vi "Coefficients for Exponential Averaging.vi"(2 "sampling frequency [Hz]":dbl=10000.0 format="%.2f", 3 "time constant [ms]":dbl=125.0 min=0.0 format="%.2f", 4 "exponential mode":enum16{"Slow", "Fast", "Impulse", "Custom"}(ring)=enum."Fast") -> (0 "actual time constant [ms]":dbl=125.0 format="%.2f", 1 "filter coefficients":T1 {"Forward Coefficients" format="%.2f"; "Reverse Coefficients" format="%.2f"})   [LabVIEW 2017]
doc: "Generates the filter coefficients that correspond to the selected exponential mode or custom time constant."
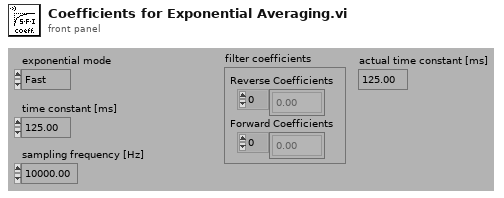
[diagram p1: front panel]
types:
  T1 = cluster{"Reverse Coefficients":dbl[], "Forward Coefficients":dbl[]}
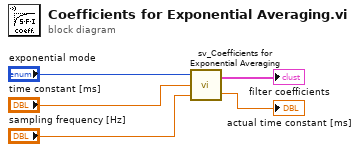
[diagram p0: block diagram]
diagram:
  n1 = call <vilib>:"sv_Coefficients for Exponential Averaging.vi"("sampling frequency [Hz]"="sampling frequency [Hz]", "time constant [ms]"="time constant [ms]", "exponential mode"="exponential mode") -> ("actual time constant [ms]"=→"actual time constant [ms]":dbl, "filter coefficients"=→"filter coefficients":T1)
